vi "Animation Test App.vi"() -> ()   [LabVIEW 2011]
uses:
  System Tools/LVH-SystemTools.lvlib
panel:
  in  "Position":cluster{"X":dbl, "Y":dbl}
  out "Loop Count":i32
  in  "Stop Button":bool
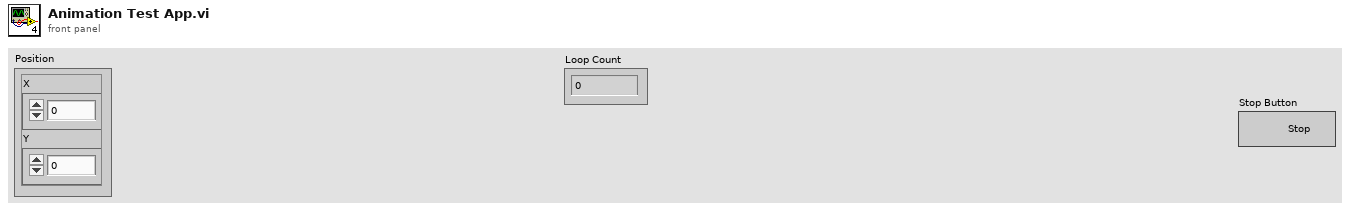
[diagram p1: front panel]
types:
  T1 = typedef "LVH-Toolbox.lvlib/LVH-SystemTools.lvlib/Animation Config.ctl" = cluster{"Image Data":T2[], "FPS":u32, "Position":cluster{"X":i16, "Y":i16}}
  T2 = typedef "imagedata.ctl" = cluster{"image type":i32, "image depth":i32, "image":u8[], "mask":u8[], "colors":u32[], "Rectangle":cluster{"left":i16, "top":i16, "right":i16, "bottom":i16}}
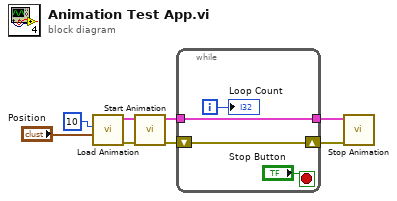
[diagram p0: block diagram]
diagram:
  n1 = call "Load Animation.vi"("Position"="Position", "FPS"=u32 10) -> ("Error Out"=w7:errorcluster, "Animation Congig"=w8:T1)  [unwired: 8 in]
  n2 = call "Start Animation.vi"("Error In"=w7, "Animation Config"=w8) -> ("Error Out"=w5:errorcluster, "Animation Config"=w6:T1)  [unwired: 8 in]
  n3 = while {
    tunnel: w6 -> [w9]
    shift-right: [w10] -> w3
    shift-left: w5 -> [w10]
    tunnel: [w9] -> w4
    i -> [w11]
    stop <- "Stop Button" stop-if-true
    "Loop Count" <- w11
  }
  n4 = call "Stop Animation.vi"("Error In"=w3, "Animation Config"=w4) -> ()  [unwired: 9 in, 1 out]
